vi "ObtainUserEvents.vi"(8 "ErrorArray":errorcluster[](array[cluster])) -> (0 "ErrorArray":errorcluster[](array[cluster]), 2 "clUserEvents":T1)   [LabVIEW 2018]
uses:
  clUserEvents.ctl
  clUserEventDataType.ctl
  <userlib>/NIST/NISTErrorLib/NISTErrorLib.lvlib
panel:
  # "DO NOT REMOVE THE STOP EVENT\n\nIf you want to add additional Request Events, open this typedef, copy an existing event and rename it to your event name."
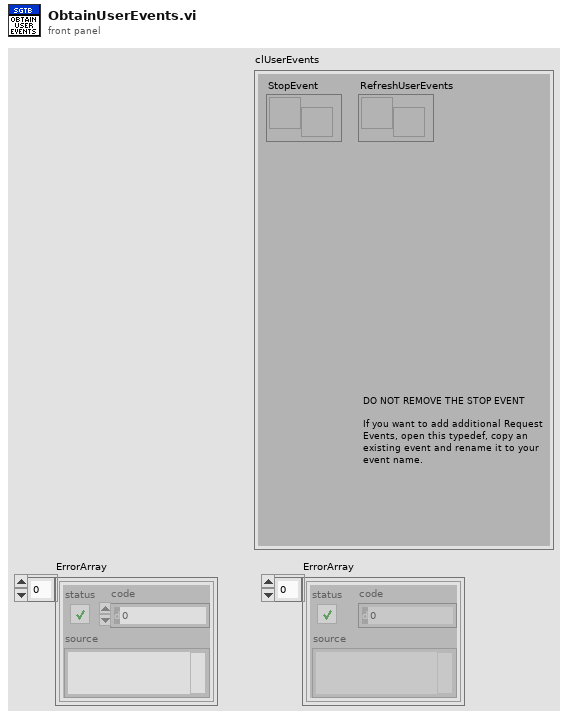
[diagram p1: front panel]
types:
  T1 = typedef "clUserEvents.ctl" = cluster{"StopEvent":refnum<user-event>, "RefreshUserEvents":refnum<user-event>}
  T2 = typedef "clUserEventDataType.ctl" = cluster{"Data":variant}
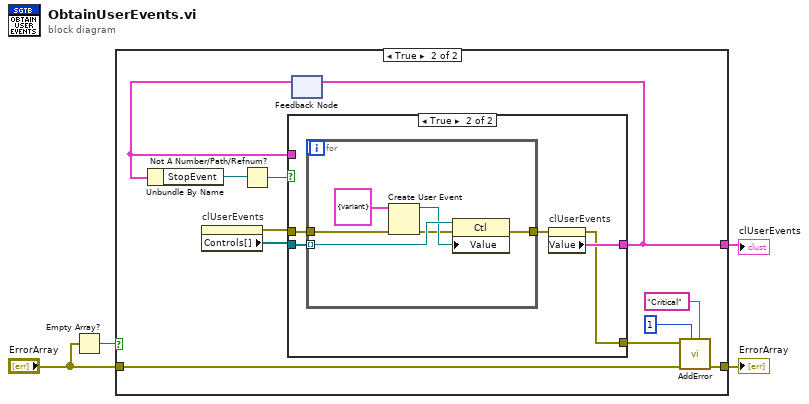
[diagram p0: block diagram]
diagram:
  n1 = Empty Array?(array="ErrorArray") -> (empty?=w2:bool)
  n2 = case shown="True" w2 {
    tunnel: [w5 w16] -> w4
    tunnel: "ErrorArray" -> [w5 w15]
    tunnel: [_ w14] -> w1
    frame False {
    }
    frame True {
      n3 = property on="clUserEvents" class="Clust (strict)"() -> (error out=w10:errorcluster, "Controls[]"=w9:refnum<vi>[])  [unwired: 2 in, 1 out]
      n4 = feedback #1() -> (w8:T1)  [unwired: 1 in]
      n5 = Unbundle By Name(w8) -> ("StopEvent"=w6:refnum<user-event>)
      n6 = Not A Number/Path/Refnum?(number/path/refnum=w6) -> (NaN/Path/Refnum?=w7:bool)
      n7 = case shown="True" w7 {
        tunnel: w9 -> [_ w21]
        tunnel: w10 -> [_ w22]
        tunnel: [w17 w19] -> w14
        tunnel: w8 -> [w17 _]
        tunnel: [_ w18] -> w13
        frame False {
        }
        frame True {
          n8 = for {
            tunnel: w22 -> [w28]
            tunnel: w21 -> [w26] mode=indexing
            tunnel: [w23] -> w20
            n9 = Create User Event(user event datatype=T2 {"Data"=variant} ("clUserEventData"), error in=w28) -> (user event=w25:refnum<user-event>, error out=w24:errorcluster)
            n10 = property class="Ctl"(reference=w26, error in=w24, "Value"=w25) -> (error out=w23:errorcluster)  [unwired: 1 out]
          }
          n11 = property on="clUserEvents" class="Clust (strict)"(error in=w20) -> (error out=w18:errorcluster, "Value"=w19:T1)  [unwired: 1 in, 1 out]
        }
      }
      n12 = feedback-in #1(w14) -> ()
      n13 = call <userlib>:"AddError.vi"("Severity"="Critical", "Priority"=u8 1, "ErrorArray"=w15, "error in (no error)"=w13) -> ("ErrorArray"=w16:errorcluster[])  [unwired: 6 in, 1 out]
    }
  }
  "ErrorArray" <- w4
  "clUserEvents" <- w1
